vi "ClusterWithBinaryStrings.vi"(0 "Cluster":T1={"Numeric"=123.0, "String"="\u0000ïÒî«¹JT\u000b‘", "String 2"="‰»¬Êÿùâ!", "String 3"="ÐÙÚ­ASDF", "String 4"="î¡¢£¤ÑÒÓÔÚÝÜÛ½", "String 5"="\u0011\u0003\u0004\u0005™4VÁÅÉÌÂáêëìäõúûÏß"}, 5 "Which Controls Are Using Default Values":bool[](array[boolean])=[FALSE, FALSE, FALSE, FALSE, FALSE, FALSE]) -> (4 "All Default Values Are Equal":bool)   [LabVIEW 2013]
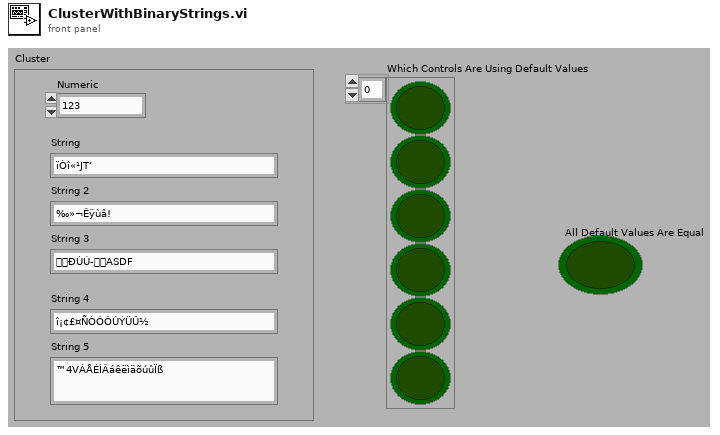
[diagram p1: front panel]
types:
  T1 = cluster{"Numeric":dbl, "String":string, "String 2":string, "String 3":string, "String 4":string, "String 5":string}
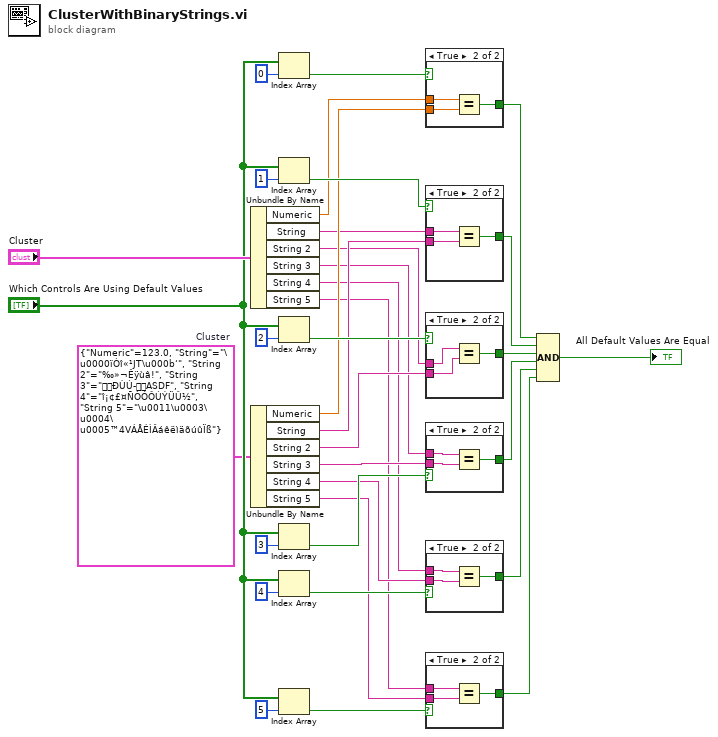
[diagram p0: block diagram]
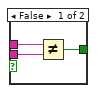
[diagram p2: hidden frame]
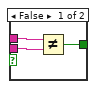
[diagram p3: hidden frame]
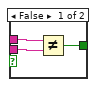
[diagram p4: hidden frame]
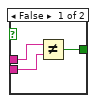
[diagram p5: hidden frame]
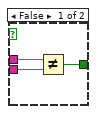
[diagram p6: hidden frame]
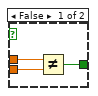
[diagram p7: hidden frame]
diagram:
  w2 = T1 {"Numeric"=123.0, "String"="\u0000ïÒî«¹JT\u000b‘", "String 2"="‰»¬Êÿùâ!", "String 3"="ÐÙÚ­ASDF", "String 4"="î¡¢£¤ÑÒÓÔÚÝÜÛ½", "String 5"="\u0011\u0003\u0004\u0005™4VÁÅÉÌÂáêëìäõúûÏß"}  # Cluster
  n1 = Unbundle By Name("Cluster") -> ("Numeric"=w26:dbl, "String"=w17:string, "String 2"=w15:string, "String 3"=w13:string, "String 4"=w11:string, "String 5"=w1:string)
  n2 = Unbundle By Name(w2) -> ("Numeric"=w25:dbl, "String"=w16:string, "String 2"=w14:string, "String 3"=w12:string, "String 4"=w10:string, "String 5"=w9:string)
  n3 = Index Array(array="Which Controls Are Using Default Values", index=0) -> (element=w32:bool)
  n4 = Index Array(array="Which Controls Are Using Default Values", index=1) -> (element=w31:bool)
  n5 = Index Array(array="Which Controls Are Using Default Values", index=2) -> (element=w30:bool)
  n6 = Index Array(array="Which Controls Are Using Default Values", index=3) -> (element=w29:bool)
  n7 = Index Array(array="Which Controls Are Using Default Values", index=4) -> (element=w28:bool)
  n8 = Index Array(array="Which Controls Are Using Default Values", index=5) -> (element=w27:bool)
  n9 = case shown="True" w32 {
    tunnel: w26 -> [w37 w40]
    tunnel: w25 -> [w36 w39]
    tunnel: [w35 w38] -> w24
    frame False {
      n10 = Not Equal?(x=w37, y=w36) -> (x != y?=w35:bool)
    }
    frame True {
      n11 = Equal?(x=w40, y=w39) -> (x = y?=w38:bool)
    }
  }
  n12 = case shown="True" w31 {
    tunnel: [w41 w46] -> w23
    tunnel: w17 -> [w43 w45]
    tunnel: w16 -> [w42 w44]
    frame False {
      n13 = Not Equal?(x=w43, y=w42) -> (x != y?=w41:bool)
    }
    frame True {
      n14 = Equal?(x=w45, y=w44) -> (x = y?=w46:bool)
    }
  }
  n15 = case shown="True" w30 {
    tunnel: [w47 w52] -> w22
    tunnel: w15 -> [w49 w51]
    tunnel: w14 -> [w48 w50]
    frame False {
      n16 = Not Equal?(x=w49, y=w48) -> (x != y?=w47:bool)
    }
    frame True {
      n17 = Equal?(x=w51, y=w50) -> (x = y?=w52:bool)
    }
  }
  n18 = case shown="True" w29 {
    tunnel: [w53 w58] -> w21
    tunnel: w13 -> [w55 w57]
    tunnel: w12 -> [w54 w56]
    frame False {
      n19 = Not Equal?(x=w55, y=w54) -> (x != y?=w53:bool)
    }
    frame True {
      n20 = Equal?(x=w57, y=w56) -> (x = y?=w58:bool)
    }
  }
  n21 = case shown="True" w28 {
    tunnel: [w59 w64] -> w20
    tunnel: w11 -> [w61 w63]
    tunnel: w10 -> [w60 w62]
    frame False {
      n22 = Not Equal?(x=w61, y=w60) -> (x != y?=w59:bool)
    }
    frame True {
      n23 = Equal?(x=w63, y=w62) -> (x = y?=w64:bool)
    }
  }
  n24 = case shown="True" w27 {
    tunnel: [w65 w70] -> w19
    tunnel: w1 -> [w67 w69]
    tunnel: w9 -> [w66 w68]
    frame False {
      n25 = Not Equal?(x=w67, y=w66) -> (x != y?=w65:bool)
    }
    frame True {
      n26 = Equal?(x=w69, y=w68) -> (x = y?=w70:bool)
    }
  }
  n27 = Compound Arithmetic op=AND(w24, w23, w22, w21, w20, w19) -> (→"All Default Values Are Equal":bool)
